vi "Enable parallel mode.vi"(8 "error in (no error)":errorcluster, 10 "Enable":bool, 11 "Scheduler in":refnum<class "Scheduler.lvclass">) -> (0 "error out":errorcluster, 3 "Scheduler out":refnum<class "Scheduler.lvclass">)   [LabVIEW 2020, in "TALOS.lvlib" / "Scheduler.lvlib" / "Scheduler.lvclass"]
uses:
  Scheduler.lvclass
  C:/LabVIEW Code/TALOS/talos/Father of all uServices/Father of all uServices/Father of all uServices.lvclass
  Father of all uServices/Father of all uServices/Father of all uServices.lvclass
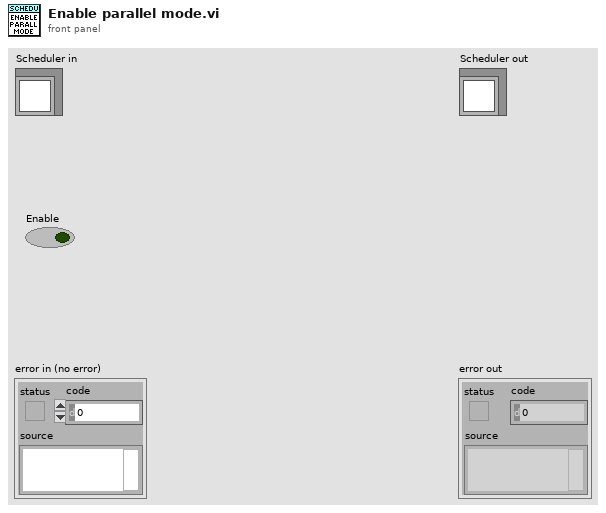
[diagram p1: front panel]
types:
  T1 = enum8{"Enabled", "Disabled", "Disabled and Grayed Out"}
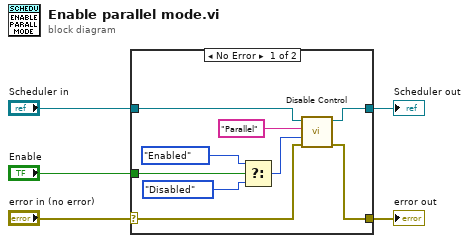
[diagram p0: block diagram]
diagram:
  n1 = case shown="No Error" "error in (no error)" {
    selector: "error in (no error)" -> [w8 w16]
    tunnel: [w6 w16] -> w4
    tunnel: [w11 w15] -> w2
    tunnel: "Scheduler in" -> [w10 w15]
    tunnel: "Enable" -> [w12 _]
    frame No Error {
      n2 = Select(t=T1."Enabled" ("Disabled"), s=w12, f=T1."Disabled" ("Disabled")) -> (s? t:f=w7:T1)
      n3 = call "Disable Control.vi"("error in (no error)"=w8, "Disabled"=w7, "FP Item Name"="Parallel", "Father of all uServices in"=w10) -> ("error out"=w6:errorcluster, "Father of all uServices out"=w11:refnum<class "Scheduler.lvclass">)  [unwired: 6 in]
    }
    frame Error {
    }
  }
  "error out" <- w4
  "Scheduler out" <- w2
